vi "Compute Distance.vi"(6 "Size Cluster":T1, 9 "Bounding Box":T2) -> (1 "Distance (ft)":dbl, 2 "Centered (output)":bool, 3 "Target Center (-1 to 1)":cluster{"X":dbl, "Y":dbl})   [LabVIEW 2011]
doc: "Using the camera lens information and the real world width of the target, determine the distance to the target."
panel:
  out "CalculatedCenterX":dbl
  out "FeetOff":dbl
  out "AngleFromHoop":dbl
  out "Ratio":dbl
  in  "Distance For Accuracy":dbl
  out "Top Vertical":bool
  out "Bottom Vertical":bool
  out "Center Vertical":bool
  out "Left Horizontal":bool
  out "Right Horizontal":bool
  out "Center Horizontal":bool
  in  "Y Image Resolution":i32
  in  "Camera view angle":dbl[](array[numeric])=[48.0, 43.5]
  in  "X Image Resolution":i32
  # "Axis 206\nAxis M1011"
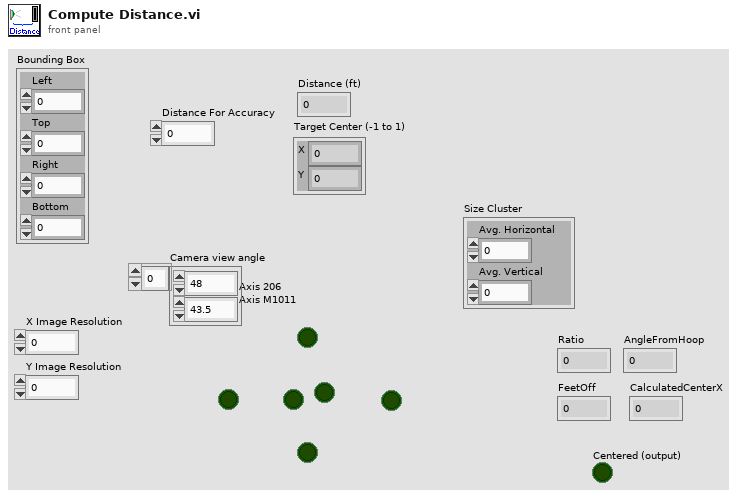
[diagram p1: front panel]
types:
  T1 = cluster{"Avg. Horizontal":dbl, "Avg. Vertical":dbl}
  T2 = cluster{"Left":dbl, "Top":dbl, "Right":dbl, "Bottom":dbl}
  T3 = cluster{"X Image Resolution":i32, "Y Image Resolution":i32}
  T4 = cluster{"X Image Resolution":dbl, "Y Image Resolution":dbl}
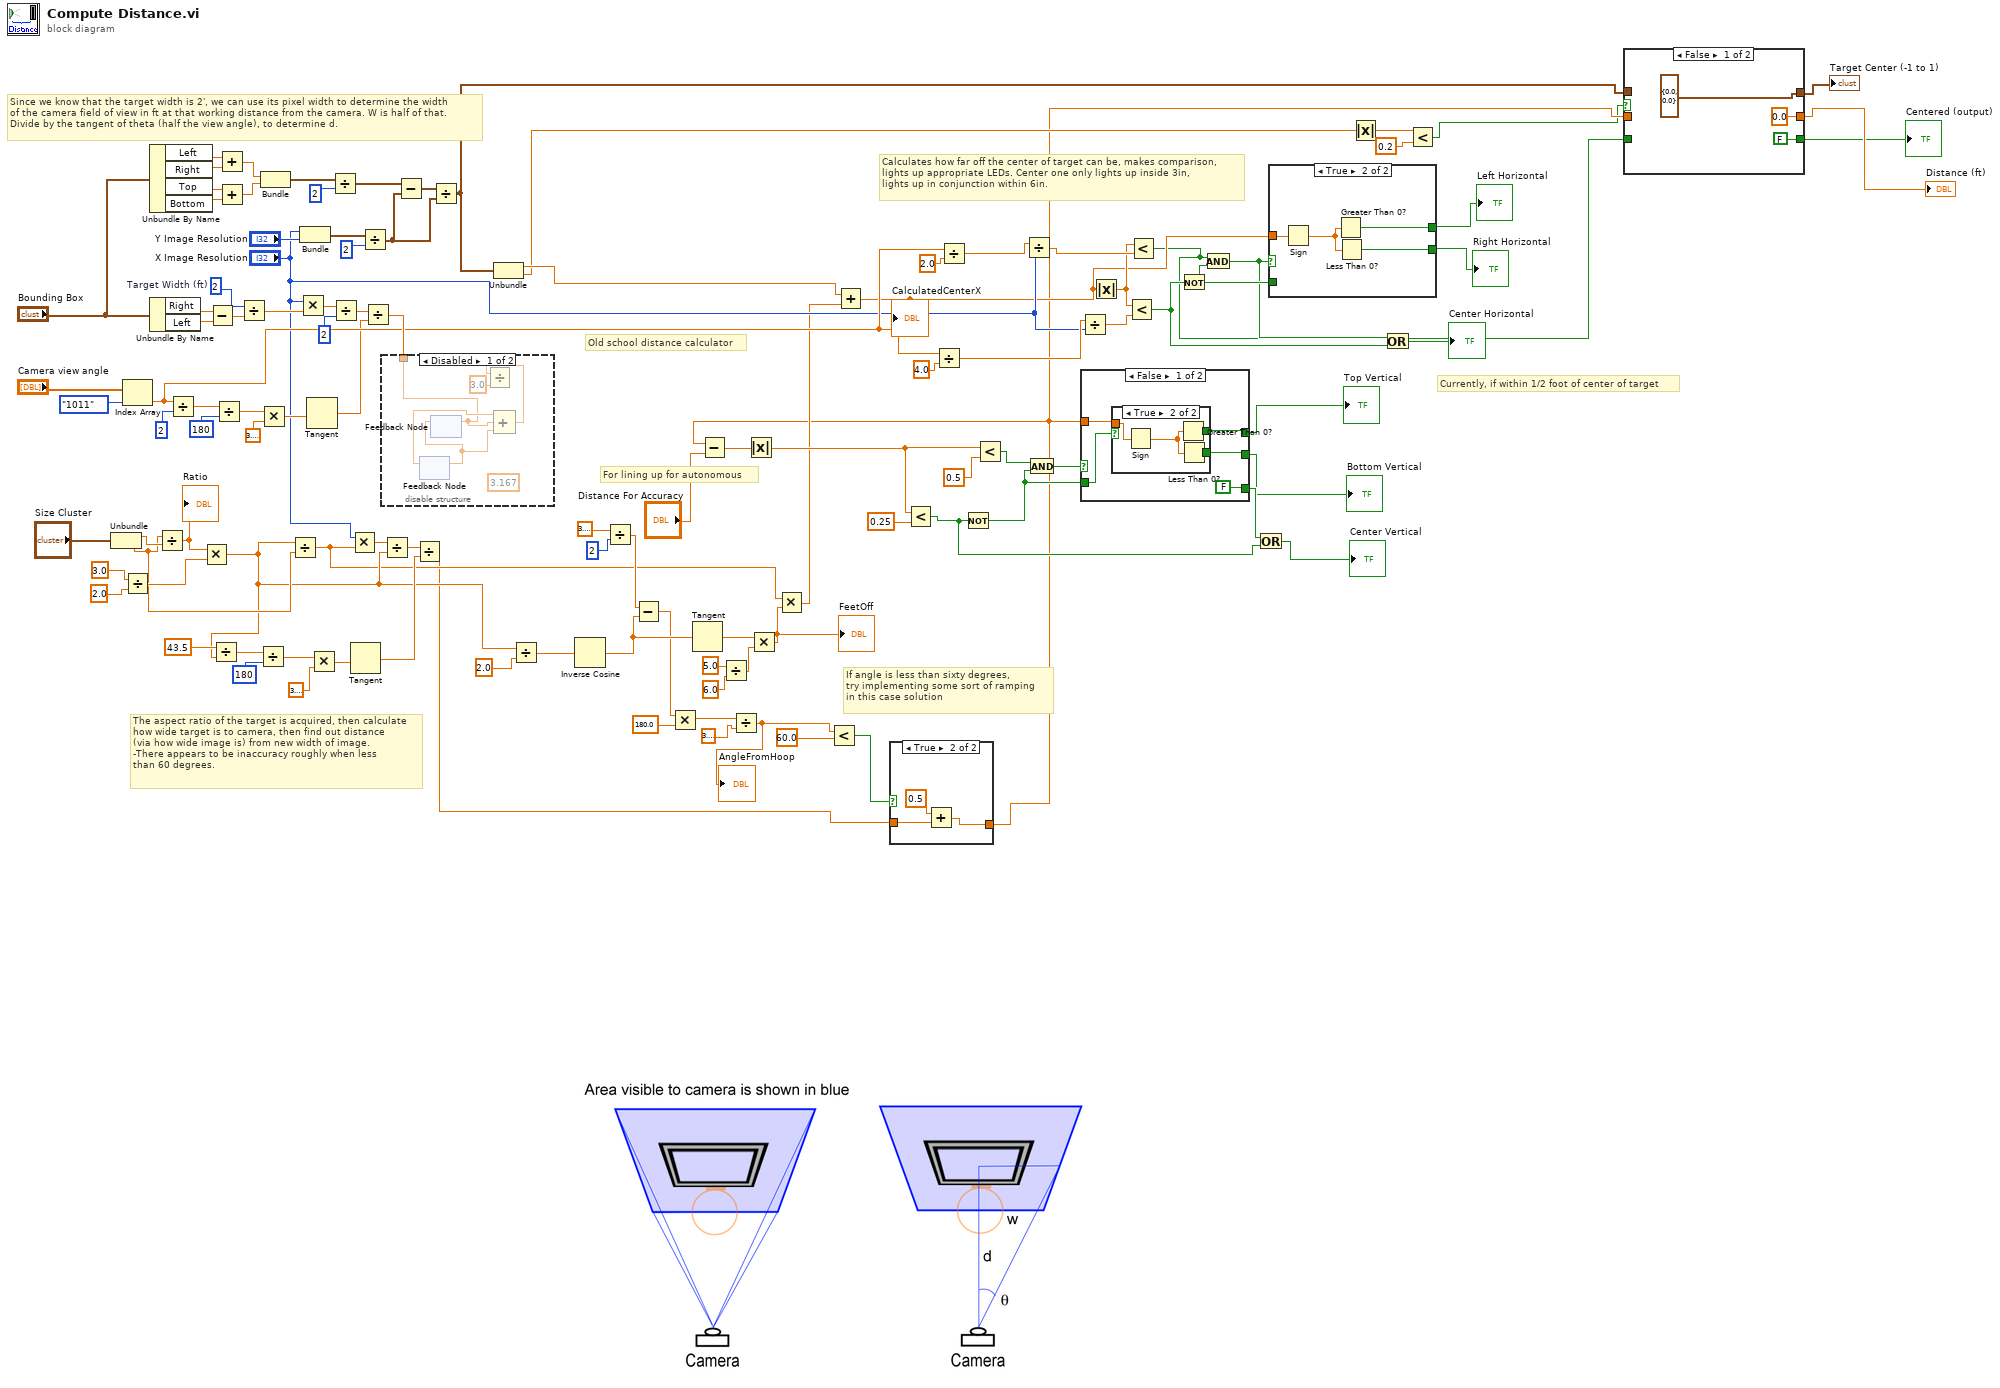
[diagram p0: block diagram]
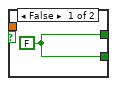
[diagram p5: hidden frame]
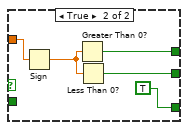
[diagram p6: hidden frame]
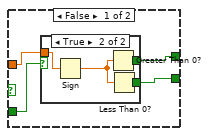
[diagram p7: hidden frame]
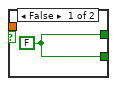
[diagram p8: hidden frame]
diagram:
  w99 = 2  # Target Width (ft)
  # "Currently, if within 1/2 foot of center of target"
  # "Calculates how far off the center of target can be, makes comparison,\nlights up appropriate LEDs. Center one only lights up inside 3in,\nlights up in conjunction within 6in."
  # "For lining up for autonomous"
  # "Old school distance calculator"
  # "The aspect ratio of the target is acquired, then calculate\nhow wide target is to camera, then find out distance \n(via how wide image is) from new width of image. \n-There appears to be inaccuracy roughly when less\nthan 60 degrees."
  # "If angle is less than sixty degrees,\ntry implementing some sort of ramping\nin this case solution"
  # "Since we know that the target width is 2', we can use its pixel width to determine the width\nof the camera field of view in ft at that working distance from the camera. W is half of that.\nDivide by the tangent of theta (half the view angle), to determine d."
  n1 = Unbundle("Size Cluster") -> ("Avg. Horizontal"=w54:dbl, "Avg. Vertical"=w39:dbl)
  n2 = Index Array(array="Camera view angle", index=enum16{"206", "1011"}."1011" ("Camera Type")) -> (element=w57:dbl)
  n3 = Divide(x=3.0, y=2.0) -> (x/y=w47:dbl)
  n4 = Unbundle By Name("Bounding Box") -> ("Left"=w94:dbl, "Right"=w95:dbl, "Top"=w97:dbl, "Bottom"=w96:dbl)
  n5 = Unbundle By Name("Bounding Box") -> ("Right"=w52:dbl, "Left"=w51:dbl)
  n6 = Divide(x=w39, y=w54) -> (x/y=w55:dbl)
  "Ratio" <- w55
  n7 = Divide(x=w57, y=2) -> (x/y=w107:dbl)
  n8 = Multiply(x=w55, y=w47) -> (x*y=w26:dbl)
  n9 = Subtract(x=w52, y=w51) -> (x-y=w101:dbl)
  n10 = Divide(x=43.5 ("y"), y=w26) -> (x/y=w44:dbl)
  n11 = Divide(x=w107, y=180) -> (x/y=w106:dbl)
  n12 = Add(x=w94, y=w95) -> (x+y=w92:dbl)
  n13 = Add(x=w97, y=w96) -> (x+y=w91:dbl)
  n14 = Divide(x=w99, y=w101) -> (x/y=w100:dbl)
  n15 = Divide(x=w44, y=180) -> (x/y=w45:dbl)
  n16 = Multiply(x=w106, y=3.141592653589793) -> (x*y=w108:dbl)
  n17 = Bundle(w92, w91) -> (w87:cluster{dbl, dbl})  [unwired: 1 in]
  n18 = Divide(x=w26, y=w39) -> (x/y=w21:dbl)
  n19 = Multiply(x="X Image Resolution", y=w100) -> (x*y=w102:dbl)
  n20 = Bundle("X Image Resolution"="X Image Resolution", "Y Image Resolution"="Y Image Resolution") -> (w89:T3)  [unwired: 1 in]
  n21 = Tangent(1:w108) -> (0:w50:dbl)
  n22 = Multiply(x=w45, y=3.141592653589793) -> (x*y=w43:dbl)
  n23 = Divide(x=w87, y=2) -> (x/y=w86:cluster{dbl, dbl})
  n24 = Divide(x=w102, y=2) -> (x/y=w104:dbl)
  n25 = Multiply(x="X Image Resolution", y=w21) -> (x*y=w20:dbl)
  n26 = Tangent(1:w43) -> (0:w41:dbl)
  n27 = Divide(x=w89, y=2) -> (x/y=w84:T4)
  n28 = Divide(x=w104, y=w50) -> (x/y=w83:dbl)
  n29 = disable-structure shown="Disabled" {
    disable-tunnel: w83 -> [w113 _]
    frame Disabled {
      (unwired) 3.167 ("y")
      n30 = feedback #1() -> (w114:dbl)  [unwired: 1 in]
      n31 = feedback #2() -> (w112:dbl)  [unwired: 1 in]
      n32 = feedback-in #1(w112) -> ()
      n33 = feedback-in #2(w113) -> ()
      n34 = Compound Arithmetic op=ADD(w114, w113, w112) -> (w115:dbl)
      n35 = Divide(x=w115, y=3.0) -> ()  [unwired: 1 out]
    }
    frame Enabled {
    }
  }
  n36 = Divide(x=w20, y=w26) -> (x/y=w53:dbl)
  n37 = Subtract(x=w86, y=w84) -> (x-y=w85:cluster{dbl, dbl})
  n38 = Divide(x=w53, y=w41) -> (x/y=w11:dbl)
  n39 = Divide(x=w85, y=w84) -> (x/y=w7:cluster{dbl, dbl})
  n40 = Unbundle(w7) -> (w19:dbl, w10:dbl)
  n41 = Divide(x=w26, y=2.0 ("x")) -> (x/y=w35:dbl)
  n42 = Inverse Cosine(1:w35) -> (0:w29:dbl)
  n43 = Divide(x=3.141592653589793, y=2) -> (x/y=w34:dbl)
  n44 = Subtract(x=w34, y=w29) -> (x-y=w22:dbl)
  n45 = Multiply(x=w22, y=180.0) -> (x*y=w23:dbl)
  n46 = Tangent(1:w29) -> (0:w28:dbl)
  n47 = Divide(x=5.0, y=6.0) -> (x/y=w32:dbl)
  n48 = Divide(x=w23, y=3.141592653589793) -> (x/y=w14:dbl)
  "AngleFromHoop" <- w14
  n49 = Multiply(x=w28, y=w32) -> (x*y=w17:dbl)
  "FeetOff" <- w17
  n50 = Multiply(x=w21, y=w17) -> (x*y=w16:dbl)
  n51 = Less?(x=w14, y=60.0) -> (x < y?=w12:bool)
  n52 = Add(x=w19, y=w16) -> (x+y=w18:dbl)
  "CalculatedCenterX" <- w18
  n53 = case shown="True" w12 {
    tunnel: w11 -> [w117 w120]
    tunnel: [w117 w118] -> w5
    frame False {
    }
    frame True {
      n54 = Add(x=0.5, y=w120) -> (x+y=w118:dbl)
    }
  }
  n55 = Subtract(x=w5, y="Distance For Accuracy") -> (x-y=w76:dbl)
  n56 = Absolute Value(x=w76) -> (abs(x)=w78:dbl)
  n57 = Less?(x=w78, y=0.25) -> (x < y?=w82:bool)
  n58 = Divide(x=w57, y=4.0) -> (x/y=w70:dbl)
  n59 = Divide(x=w57, y=2.0) -> (x/y=w72:dbl)
  n60 = Not(x=w82) -> (.not. x?=w68:bool)
  n61 = Less?(x=w78, y=0.5) -> (x < y?=w80:bool)
  n62 = Divide(x=w72, y="X Image Resolution") -> (x/y=w73:dbl)
  n63 = And(x=w80, y=w68) -> (x .and. y?=w62:bool)
  n64 = Divide(x=w70, y="X Image Resolution") -> (x/y=w58:dbl)
  n65 = case shown="False" w62 {
    tunnel: [w124 w134] -> w60
    tunnel: [w123 w133] -> w61
    tunnel: w5 -> [w125 w132]
    tunnel: w68 -> [w122 _]
    tunnel: [FALSE TRUE] -> w75
    frame False {
      n66 = case shown="True" w122 {
        tunnel: [w126 w129] -> w124
        tunnel: w125 -> [_ w128]
        tunnel: [w126 w127] -> w123
        frame False {
          w126 = FALSE
        }
        frame True {
          n67 = Sign(1:w128) -> (0:w130:dbl)
          n68 = Greater Than 0?(x=w130) -> (x > 0?=w129:bool)
          n69 = Less Than 0?(x=w130) -> (x < 0?=w127:bool)
        }
      }
    }
    frame True {
      n70 = Sign(1:w132) -> (0:w135:dbl)
      n71 = Greater Than 0?(x=w135) -> (x > 0?=w134:bool)
      n72 = Less Than 0?(x=w135) -> (x < 0?=w133:bool)
    }
  }
  "Bottom Vertical" <- w61
  "Top Vertical" <- w60
  n73 = Absolute Value(x=w18) -> (abs(x)=w59:dbl)
  n74 = Less?(x=w59, y=w58) -> (x < y?=w66:bool)
  n75 = Less?(x=w59, y=w73) -> (x < y?=w3:bool)
  n76 = Not(x=w66) -> (.not. x?=w67:bool)
  n77 = And(x=w3, y=w67) -> (x .and. y?=w15:bool)
  n78 = Or(x=w75, y=w82) -> (x .or. y?=→"Center Vertical":bool)
  n79 = case shown="True" w15 {
    tunnel: w18 -> [w137 w148]
    tunnel: [w138 w146] -> w63
    tunnel: [w136 w145] -> w64
    tunnel: w67 -> [w139 _]
    frame False {
      n80 = case shown="True" w139 {
        tunnel: [w140 w143] -> w138
        tunnel: w137 -> [_ w142]
        tunnel: [w140 w141] -> w136
        frame False {
          w140 = FALSE
        }
        frame True {
          n81 = Sign(1:w142) -> (0:w144:dbl)
          n82 = Greater Than 0?(x=w144) -> (x > 0?=w143:bool)
          n83 = Less Than 0?(x=w144) -> (x < 0?=w141:bool)
        }
      }
    }
    frame True {
      n84 = Sign(1:w148) -> (0:w147:dbl)
      n85 = Greater Than 0?(x=w147) -> (x > 0?=w146:bool)
      n86 = Less Than 0?(x=w147) -> (x < 0?=w145:bool)
    }
  }
  "Right Horizontal" <- w64
  "Left Horizontal" <- w63
  n87 = Absolute Value(x=w10) -> (abs(x)=w9:dbl)
  n88 = Or(x=w15, y=w66) -> (x .or. y?=→"Center Horizontal":bool)
  n89 = Less?(x=w9, y=0.2) -> (x < y?=w1:bool)
  n90 = case shown="False" w1 {
    tunnel: w3 -> [_ w152]
    tunnel: w5 -> [_ w153]
    tunnel: w7 -> [_ w154]
    tunnel: [cluster{dbl, dbl} {0.0, 0.0} w154] -> w6
    tunnel: [0.0 w153] -> w4
    tunnel: [FALSE w152] -> w2
    frame False {
    }
    frame True {
    }
  }
  "Distance (ft)" <- w4
  "Target Center (-1 to 1)" <- w6
  "Centered (output)" <- w2
